vi "Guidance_1.vi"(7 "Guidance gains":dbl[][](array[numeric]), 8 "k_acc":cluster{"lat_acc_mod":dbl, "up_acc":dbl}, 9 "Position (i+1)":T1, 10 "Time":T2, 11 "Data":dbl[][](array[numeric])) -> (0 "e(i+1)":dbl[](array[numeric]), 2 "new_ref[deg]":cluster{"phi":dbl, "theta":dbl, "psi":dbl})   [LabVIEW 2017]
uses:
  <vilib>/Analysis/coordinate.llb/Euler Rotation Order.ctl
  <vilib>/Analysis/NI_AALPro.lvlib
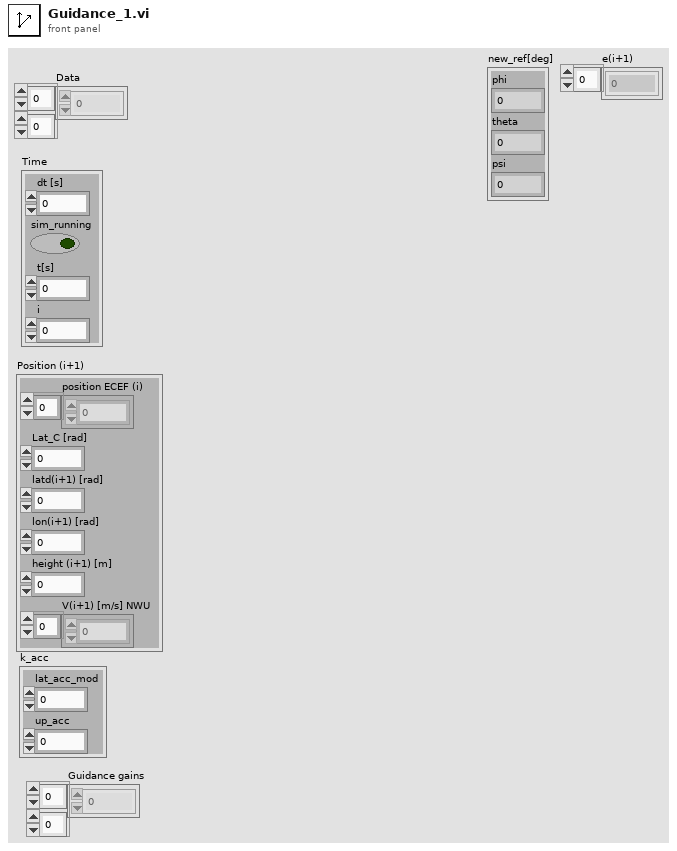
[diagram p1: front panel]
types:
  T1 = cluster{"position ECEF (i)":dbl[], "Lat_C [rad]":dbl, "latd(i+1) [rad]":dbl, "lon(i+1) [rad]":dbl, "height (i+1) [m]":dbl, "V(i+1) [m/s] NWU":dbl[]}
  T2 = cluster{"dt [s]":dbl, "sim_running":bool, "t[s]":dbl, "i":i32}
  T3 = typedef "NI_AALPro.lvlib/Euler Rotation Order.ctl" = u16
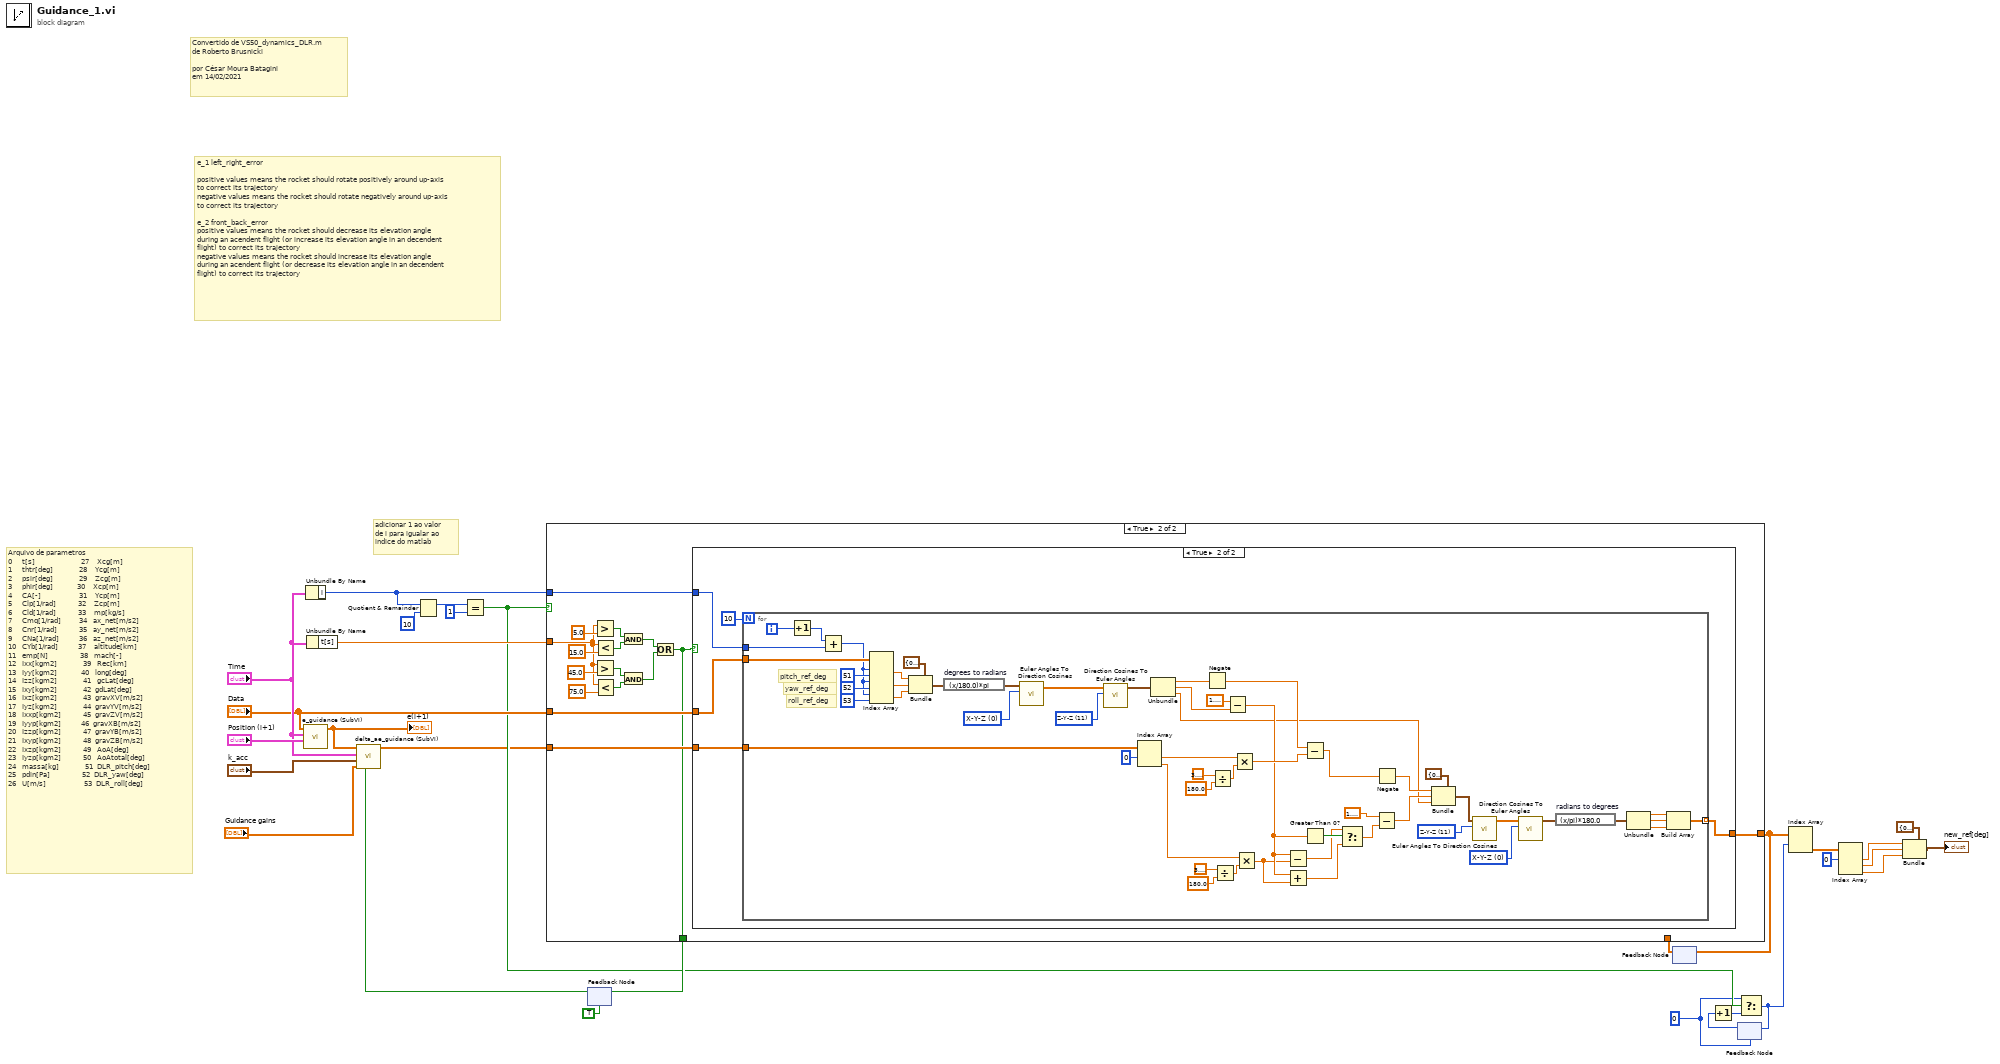
[diagram p0: block diagram]
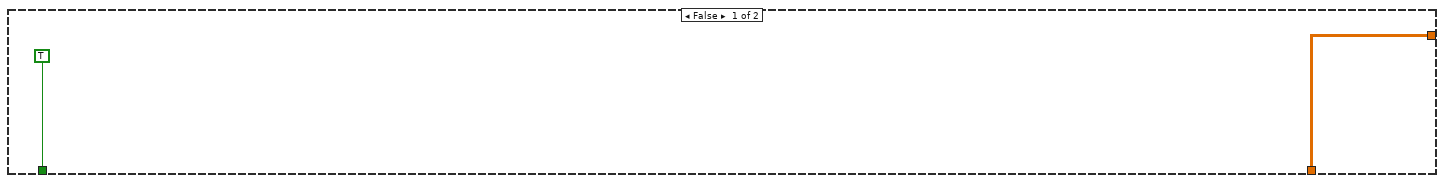
[diagram p2: hidden frame]
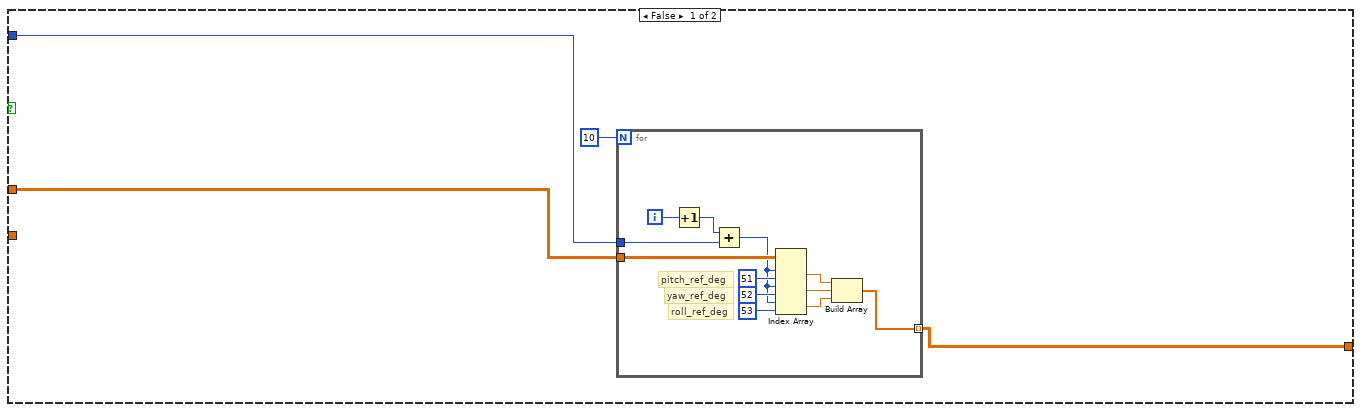
[diagram p3: hidden frame]
diagram:
  w6 = 0 ("t")
  # "adicionar 1 ao valor \nde i para igualar ao \nindice do matlab"
  # "Convertido de VS50_dynamics_DLR.m\nde Roberto Brusnicki\n\npor César Moura Batagini\nem 14/02/2021"
  # "e_1 left_right_error\n\npositive values means the rocket should rotate positively around up-axis \nto correct its trajectory\nnegative values means the rocket should rotate negatively around up-axis \nto correct its trajectory\n\ne_2 front_back_error\npositive values means the rocket should decrease its elevation angle\nduring an acendent flight (or increase its elevation angle in an decendent \nflight) to correct its trajectory\nnegative values means the rocket should increase its elevation angle\nduring an acendent flight (or decrease its elevation angle in an decendent \nflight) to correct its trajectory"
  # "Arquivo de parametros\n0     t[s]                       27    Xcg[m] \n1     thtr[deg]             28    Ycg[m]\n2     psir[deg]             29    Zcg[m]  \n3     phir[deg]            30    Xcp[m]       \n4     CA[-]                   31    Ycp[m]        \n5     Clp[1/rad]           32    Zcp[m]     \n6     Cld[1/rad]           33    mp[kg/s]        \n7     Cmq[1/rad]         34   ax_net[m/s2]         \n8     Cnr[1/rad]           35   ay_net[m/s2]      \n9     CNa[1/rad]          36   az_net[m/s2]      \n10   CYb[1/rad]          37    altitude[km]       \n11   emp[N]                38   mach[-]     \n12   Ixx[kgm2]             39   Rec[km]     \n13   Iyy[kgm2]            40   long[deg]     \n14   Izz[kgm2]             41   gcLat[deg]        \n15   Ixy[kgm2]             42  gdLat[deg]       \n16   Ixz[kgm2]             43  gravXV[m/s2]  \n17   Iyz[kgm2]             44  gravYV[m/s2]     \n18   Ixxp[kgm2]           45  gravZV[m/s2]         \n19   Iyyp[kgm2]          46  gravXB[m/s2]         \n20   Izzp[kgm2]           47  gravYB[m/s2]         \n21   Ixyp[kgm2]           48  gravZB[m/s2]           \n22   Ixzp[kgm2]           49   AoA[deg]             \n23   Iyzp[kgm2]           50   AoAtotal[deg]       \n24   massa[kg]             51  DLR_pitch[deg]    \n25   pdin[Pa]                52  DLR_yaw[deg]  \n26   U[m/s]                   53  DLR_roll[deg]"
  n1 = call "e_guidance (SubVI).vi"("Position (i+1)"="Position (i+1)", "Time"="Time", "Data"="Data") -> ("e(i+1)"=w27:dbl[])  [unwired: 8 in]
  "e(i+1)" <- w27
  n2 = Unbundle By Name("Time") -> ("i"=w7:i32)
  n3 = Unbundle By Name("Time") -> ("t[s]"=w22:dbl)
  n4 = Quotient & Remainder(x=w7, y=10) -> (x-y*floor(x/y)=w25:i32)  [unwired: 1 out]
  n5 = Equal?(x=w25, y=1) -> (x = y?=w8:bool)
  n6 = feedback #1(TRUE) -> (w20:bool)
  n7 = call "delta_ae_guidance (SubVI).vi"("Boolean"=w20, "Guidance gains"="Guidance gains", "k_acc"="k_acc", "Time"="Time", "e(i+1)"=w27) -> ("Delta azi_ele"=w2:dbl[])  [unwired: 6 in]
  n8 = feedback #2() -> (w9:dbl[][])  [unwired: 1 in]
  n9 = case shown="True" w8 {
    tunnel: w22 -> [_ w38]
    tunnel: w7 -> [_ w36]
    tunnel: "Data" -> [_ w35]
    tunnel: w2 -> [_ w34]
    tunnel: [TRUE w32] -> w18
    tunnel: [w30 w33] -> w10
    tunnel: w9 -> [w30 _]
    frame False {
    }
    frame True {
      n10 = Greater?(x=w38, y=5.0) -> (0:w46:bool)
      n11 = Greater?(x=w38, y=45.0) -> (0:w40:bool)
      n12 = Less?(x=w38, y=15.0) -> (x < y?=w47:bool)
      n13 = Less?(x=w38, y=75.0) -> (x < y?=w39:bool)
      n14 = And(x=w46, y=w47) -> (x .and. y?=w43:bool)
      n15 = And(x=w40, y=w39) -> (x .and. y?=w37:bool)
      n16 = Or(x=w43, y=w37) -> (x .or. y?=w32:bool)
      n17 = case shown="True" w32 {
        tunnel: w36 -> [w50 w67]
        tunnel: w35 -> [w49 w66]
        tunnel: w34 -> [_ w65]
        tunnel: [w48 w64] -> w33
        frame False {
          n18 = for {
            N: 10 -> [_]
            tunnel: w50 -> [w59]
            tunnel: w49 -> [w58]
            tunnel: [w52] -> w48 mode=indexing
            i -> [w56]
            # "roll_ref_deg"
            # "yaw_ref_deg"
            # "pitch_ref_deg"
            n19 = Increment(x=w56) -> (x+1=w60:i32)
            n20 = Add(x=w60, y=w59) -> (x+y=w57:i32)
            n21 = Index Array(array=w58, index (row) #1=w57, index (col) #1=51 ("disabled index (col)"), index (row) #2=w57, index (col) #2=52 ("disabled index (col)"), index (row) #3=w57, index (col) #3=53 ("disabled index (col)")) -> (element #1=w55:dbl, element #2=w54:dbl, element #3=w53:dbl)
            n22 = Build Array(w55, w54, w53) -> (w52:dbl[])
          }
        }
        frame True {
          n23 = for {
            N: 10 -> [_]
            tunnel: w67 -> [w102]
            tunnel: w66 -> [w116]
            tunnel: w65 -> [w69]
            tunnel: [w70] -> w64 mode=indexing
            i -> [w77]
            w81 = T3 0 items=["X-Y-Z", "X-Z-Y", "Y-X-Z", "Y-Z-X", "Z-X-Y", "Z-Y-X", "X-Y-X", "X-Z-X", "Y-X-Y", "Y-Z-Y", "Z-X-Z", "Z-Y-Z"] ("rotation order")
            w82 = T3 11 items=["X-Y-Z", "X-Z-Y", "Y-X-Z", "Y-Z-X", "Z-X-Y", "Z-Y-X", "X-Y-X", "X-Z-X", "Y-X-Y", "Y-Z-Y", "Z-X-Z", "Z-Y-Z"] ("rotation order")
            w113 = T3 11 items=["X-Y-Z", "X-Z-Y", "Y-X-Z", "Y-Z-X", "Z-X-Y", "Z-Y-X", "X-Y-X", "X-Z-X", "Y-X-Y", "Y-Z-Y", "Z-X-Z", "Z-Y-Z"] ("rotation order")
            w115 = T3 0 items=["X-Y-Z", "X-Z-Y", "Y-X-Z", "Y-Z-X", "Z-X-Y", "Z-Y-X", "X-Y-X", "X-Z-X", "Y-X-Y", "Y-Z-Y", "Z-X-Z", "Z-Y-Z"] ("rotation order")
            # "roll_ref_deg"
            # "yaw_ref_deg"
            # "pitch_ref_deg"
            n24 = Increment(x=w77) -> (x+1=w103:i32)
            n25 = Add(x=w103, y=w102) -> (x+y=w78:i32)
            n26 = Index Array(array=w116, index (row) #1=w78, index (col) #1=51 ("disabled index (col)"), index (row) #2=w78, index (col) #2=52 ("disabled index (col)"), index (row) #3=w78, index (col) #3=53 ("disabled index (col)")) -> (element #1=w119:dbl, element #2=w118:dbl, element #3=w117:dbl)
            n27 = Bundle(cluster=cluster{"phi":dbl, "theta":dbl, "psi":dbl} {"phi"=0.0, "theta"=0.0, "psi"=0.0} ("Euler Angles"), "phi"=w119, "theta"=w118, "psi"=w117) -> (w76:cluster{"phi":dbl, "theta":dbl, "psi":dbl})
            n28 = expression code="(x/180.0)*pi" "degrees to radians"(w76) -> (w75:cluster{"phi":dbl, "theta":dbl, "psi":dbl})
            n29 = call <vilib>:"Euler Angles To Direction Cosines.vi"("rotation order"=w115, "Euler Angles"=w75) -> ("Direction Cosines"=w114:dbl[][])  [unwired: 8 in, 1 out]
            n30 = call <vilib>:"Direction Cosines To Euler Angles.vi"("rotation order"=w113, "Direction Cosines"=w114) -> ("Euler Angles"=w112:cluster{"phi":dbl, "theta":dbl, "psi":dbl})  [unwired: 8 in, 1 out]
            n31 = Index Array(array=w69, index #1=0 ("index")) -> (element #1=w104:dbl, element #2=w95:dbl)  [unwired: 1 in]
            n32 = Unbundle(w112) -> ("phi"=w109:dbl, "theta"=w110:dbl, "psi"=w83:dbl)
            n33 = Negate(x=w109) -> (-x=w101:dbl)
            n34 = Divide(x=3.141592653589793, y=180.0) -> (x/y=w106:dbl)
            n35 = Divide(x=3.141592653589793, y=180.0) -> (x/y=w98:dbl)
            n36 = Subtract(x=1.5707963267948966, y=w110) -> (x-y=w93:dbl)
            n37 = Multiply(x=w104, y=w106) -> (x*y=w100:dbl)
            n38 = Multiply(x=w95, y=w98) -> (x*y=w92:dbl)
            n39 = Subtract(x=w93, y=w92) -> (x-y=w94:dbl)
            n40 = Add(x=w93, y=w92) -> (x+y=w91:dbl)
            n41 = Subtract(x=w101, y=w100) -> (x-y=w88:dbl)
            n42 = Greater Than 0?(x=w93) -> (x > 0?=w99:bool)
            n43 = Select(t=w94, s=w99, f=w91) -> (s? t:f=w85:dbl)
            n44 = Subtract(x=1.5707963267948966, y=w85) -> (x-y=w84:dbl)
            n45 = Negate(x=w88) -> (-x=w87:dbl)
            n46 = Bundle(cluster=cluster{"phi":dbl, "theta":dbl, "psi":dbl} {"phi"=0.0, "theta"=0.0, "psi"=0.0} ("Euler Angles"), "phi"=w87, "theta"=w84, "psi"=w83) -> (w89:cluster{"phi":dbl, "theta":dbl, "psi":dbl})
            n47 = call <vilib>:"Euler Angles To Direction Cosines.vi"("rotation order"=w82, "Euler Angles"=w89) -> ("Direction Cosines"=w80:dbl[][])  [unwired: 8 in, 1 out]
            n48 = call <vilib>:"Direction Cosines To Euler Angles.vi"("rotation order"=w81, "Direction Cosines"=w80) -> ("Euler Angles"=w79:cluster{"phi":dbl, "theta":dbl, "psi":dbl})  [unwired: 8 in, 1 out]
            n49 = expression code="(x/pi)*180.0" "radians to degrees"(w79) -> (w74:cluster{"phi":dbl, "theta":dbl, "psi":dbl})
            n50 = Unbundle(w74) -> ("phi"=w73:dbl, "theta"=w71:dbl, "psi"=w72:dbl)
            n51 = Build Array(w73, w71, w72) -> (w70:dbl[])
          }
        }
      }
    }
  }
  n52 = feedback-in #1(w18) -> ()
  n53 = feedback-in #2(w10) -> ()
  n54 = feedback #3(w6) -> (w5:i32)
  n55 = Increment(x=w5) -> (x+1=w4:i32)
  n56 = Select(t=w6, s=w8, f=w4) -> (s? t:f=w3:i32)
  n57 = feedback-in #3(w3) -> ()
  n58 = Index Array(array=w10, index (row)=w3) -> (element=w16:dbl[])  [unwired: 1 in]
  n59 = Index Array(array=w16, index #1=0 ("index")) -> (element #1=w14:dbl, element #2=w12:dbl, element #3=w13:dbl)  [unwired: 2 in]
  n60 = Bundle(cluster=cluster{"phi":dbl, "theta":dbl, "psi":dbl} {"phi"=0.0, "theta"=0.0, "psi"=0.0} ("Euler Angles"), "phi"=w14, "theta"=w12, "psi"=w13) -> (→"new_ref[deg]":cluster{"phi":dbl, "theta":dbl, "psi":dbl})
